vi "(SUBVI) - Sense Forcfe.vi"(10 "Port (Port 1)":T2=2 items=["Port 1", "Port 2", "Port 3", "Port 4"], 11 "NXT/EV3":T1) -> (1 "raw dif":dbl, 3 "NXT/EV3 2":T1, 9 "Scaled dif":dbl)   [LabVIEW 2016]
uses:
  <vilib>/NXT/Subs/LVHSConnector.ctl
  <vilib>/NXT/LegoClasses/BrickReference/BrickReference.lvclass
  <vilib>/NXT/Block Support/NXT_InputPort.ctl
  <vilib>/NXT/Block Support/NXT_OutputPort.ctl
  testrobot.lvrbt
panel:
  out "Raw Value 2":i16=2550
  out "Scaled Value 2":i16=387
  out "Raw Value":i16=2550
  out "Scaled Value":i16=387
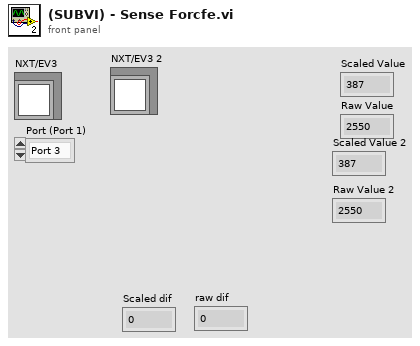
[diagram p1: front panel]
types:
  T1 = typedef "LVHSConnector.ctl" = refnum<class "BrickReference.lvclass">
  T2 = typedef "NXT_InputPort.ctl" = u32
  T3 = typedef "NXT_OutputPort.ctl" = u8
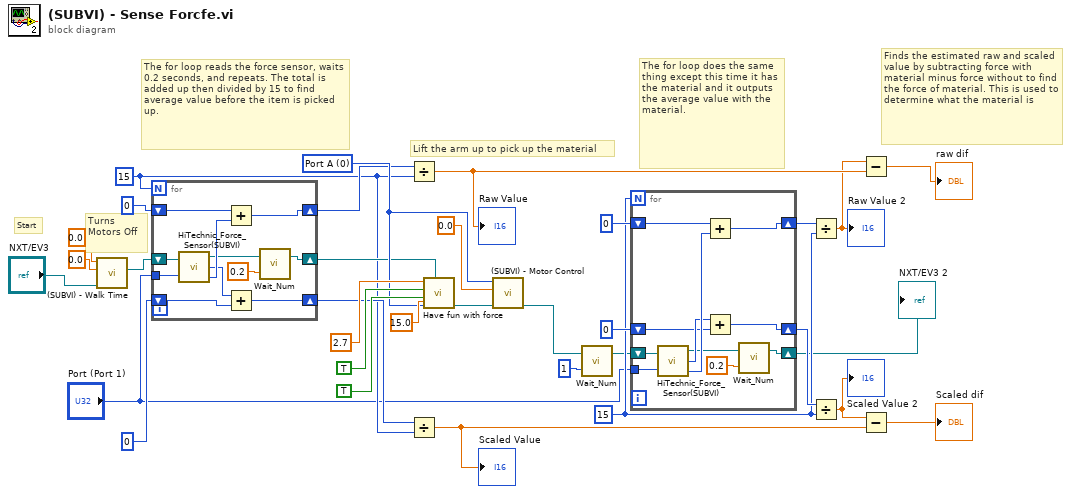
[diagram p0: block diagram]
diagram:
  w10 = 15
  w15 = 15
  w29 = T3 0 items=["Port A", "Port B", "Port C", "Port D"] ("Motors")
  # "Finds the estimated raw and scaled value by subtracting force with material minus force without to find the force of material. This is used to determine what the material is"
  # "The for loop does the same thing except this time it has the material and it outputs the average value with the material."
  # "Lift the arm up to pick up the material"
  # "Turns Motors Off"
  # "The for loop reads the force sensor, waits 0.2 seconds, and repeats. The total is added up then divided by 15 to find average value before the item is picked up."
  # "Start"
  n1 = call "(SUBVI) - Walk Time.vi"("NXT/EV3"="NXT/EV3", "Time walking"=0.0, "Walk Speed"=0.0) -> ("NXT/EV3 2"=w4:T1)  [unwired: 8 in]
  n2 = for {
    N: w15 -> [_]
    tunnel: "Port (Port 1)" -> [w43]
    shift-right: [w35] -> w25
    shift-left: w4 -> [w44]
    shift-right: [w41] -> w19
    shift-left: 0 -> [w42]
    shift-right: [w38] -> w17
    shift-left: 0 -> [w37]
    n3 = call "HiTechnic_Force_Sensor(SUBVI).vi"("NXT/EV3"=w44, "Port (Port 1)"=w43) -> ("NXT/EV3"=w36:T1, "Scaled Value"=w39:i16, "Raw Value"=w40:i16)
    n4 = Add(x=w42, y=w40) -> (x+y=w41:i32)
    n5 = Add(x=w39, y=w37) -> (x+y=w38:i32)
    n6 = call <vilib>:"Wait_Num.vi"("Time (1 sec)"=0.2, "NXT/EV3"=w36) -> ("NXT/EV3"=w35:T1)  [unwired: 2 in]
  }
  n7 = Divide(x=w19, y=w15) -> (x/y=w18:dbl)
  "Raw Value" <- w18
  n8 = Divide(x=w17, y=w15) -> (x/y=w16:dbl)
  "Scaled Value" <- w16
  n9 = call "Have fun with force.vi"("Speed"=15.0, "NXT/EV3"=w25, "Motors"=w29, "Up/Down"=TRUE, "Run"=TRUE, "Time"=2.7) -> ("NXT/EV3 2"=w22:T1)  [unwired: 5 in]
  n10 = call "(SUBVI) - Motor Control.vi"("NXT/EV3"=w22, "Speed"=0.0, "Motors"=w29) -> ("NXT/EV3 2"=w27:T1)  [unwired: 8 in]
  n11 = call <vilib>:"Wait_Num.vi"("Time (1 sec)"=1, "NXT/EV3"=w27) -> ("NXT/EV3"=w9:T1)  [unwired: 2 in]
  n12 = for {
    N: w10 -> [_]
    tunnel: "Port (Port 1)" -> [w54]
    shift-right: [w46] -> w1
    shift-left: w9 -> [w55]
    shift-right: [w52] -> w12
    shift-left: 0 -> [w53]
    shift-right: [w49] -> w11
    shift-left: 0 -> [w48]
    n13 = call "HiTechnic_Force_Sensor(SUBVI).vi"("NXT/EV3"=w55, "Port (Port 1)"=w54) -> ("NXT/EV3"=w47:T1, "Scaled Value"=w50:i16, "Raw Value"=w51:i16)
    n14 = Add(x=w53, y=w51) -> (x+y=w52:i32)
    n15 = Add(x=w50, y=w48) -> (x+y=w49:i32)
    n16 = call <vilib>:"Wait_Num.vi"("Time (1 sec)"=0.2, "NXT/EV3"=w47) -> ("NXT/EV3"=w46:T1)  [unwired: 2 in]
  }
  "NXT/EV3 2" <- w1
  n17 = Divide(x=w12, y=w10) -> (x/y=w6:dbl)
  "Raw Value 2" <- w6
  n18 = Divide(x=w11, y=w10) -> (x/y=w7:dbl)
  "Scaled Value 2" <- w7
  n19 = Subtract(x=w6, y=w18) -> (x-y=→"raw dif":dbl)
  n20 = Subtract(x=w7, y=w16) -> (x-y=→"Scaled dif":dbl)
